vi "Find Channel Names Array.vi"(11 "Instrument Driver Method Descriptor Array":T2) -> (1 "Found?":bool, 2 "Channel List Size":i32, 3 "Channel Names":T1)   [LabVIEW 2021]
uses:
  <vilib>/myRIO/Common/Express VI Framework/typedefs/Instrument Driver Method Descriptor Array.ctl
  <vilib>/myRIO/Common/Express VI Framework/typedefs/Instrument Driver Method Descriptor.ctl
  <vilib>/myRIO/Common/Express VI Framework/typedefs/Channel Alias List.ctl
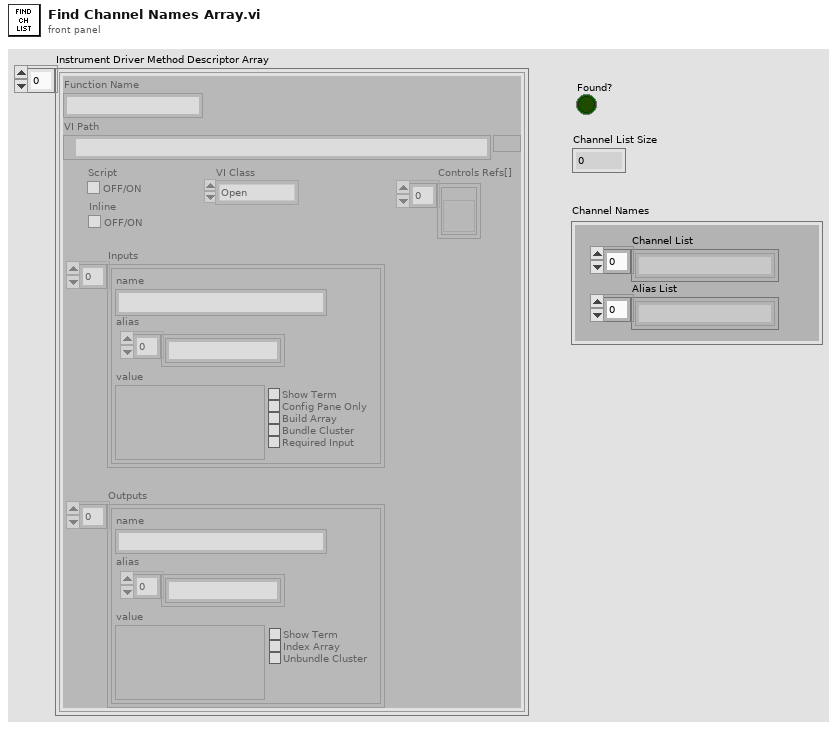
[diagram p1: front panel]
types:
  T1 = typedef "Channel Alias List.ctl" = cluster{"Channel List":string[], "Alias List":string[]}
  T2 = typedef "Instrument Driver Method Descriptor Array.ctl" = T3[]
  T3 = typedef "Instrument Driver Method Descriptor.ctl" = cluster{"Function Name":string, "VI Path":path, "Script":bool, "Inputs":cluster{"name":string, "value":variant, "Config Pane Only":bool, "Build Array":bool, "Bundle Cluster":bool, "Show Term":bool, "alias":string[], "Required Input":bool}[], "Outputs":cluster{"name":string, "value":variant, "Show Term":bool, "Index Array":bool, "Unbundle Cluster":bool, "alias":string[]}[], "VI Class":enum16{"Open", "Configure", "Data", "Manage", "Close"}, "Controls Refs[]":refnum<vi>[], "Inline":bool}
  T4 = cluster{"name":string, "value":variant, "Config Pane Only":bool, "Build Array":bool, "Bundle Cluster":bool, "Show Term":bool, "alias":string[], "Required Input":bool}[]
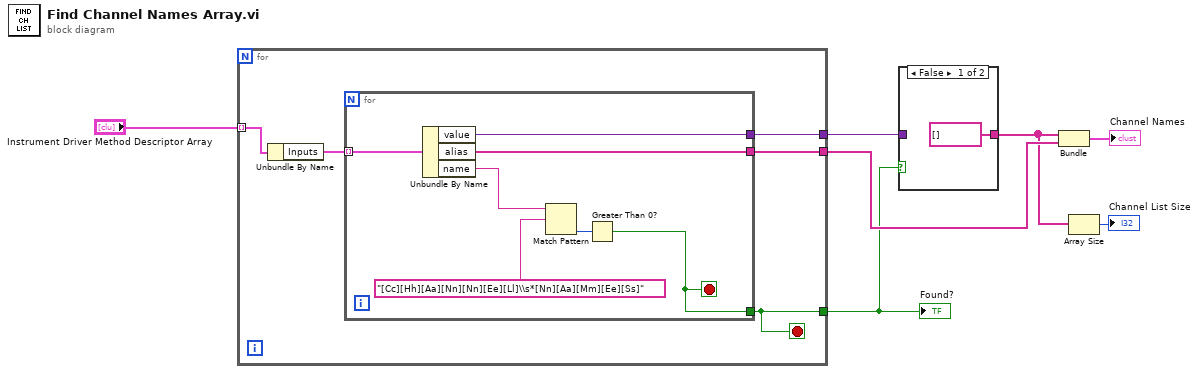
[diagram p0: block diagram]
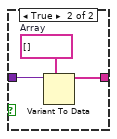
[diagram p2: hidden frame]
diagram:
  n1 = for {
    tunnel: "Instrument Driver Method Descriptor Array" -> [w12] mode=indexing
    tunnel: [w11] -> w6
    tunnel: [w10] -> w5
    tunnel: [w9] -> w1
    stop <- w9 stop-if-true
    n2 = Unbundle By Name(w12) -> ("Inputs"=w8:T4)
    n3 = for {
      tunnel: w8 -> [w16] mode=indexing
      tunnel: [w15] -> w9
      tunnel: [w14] -> w11
      tunnel: [w13] -> w10
      stop <- w15 stop-if-true
      n4 = Unbundle By Name(w16) -> ("value"=w14:variant, "alias"=w13:string[], "name"=w19:string)
      n5 = Match Pattern(string=w19, regular expression="[Cc][Hh][Aa][Nn][Nn][Ee][Ll]\\s*[Nn][Aa][Mm][Ee][Ss]") -> (offset past match=w18:i32)  [unwired: 1 in, 3 out]
      n6 = Greater Than 0?(x=w18) -> (x > 0?=w15:bool)
    }
  }
  "Found?" <- w1
  n7 = case shown="False" w1 {
    tunnel: w6 -> [_ w22]
    tunnel: [string[] [] ("Array") w21] -> w3
    frame False {
    }
    frame True {
      w23 = string[] []  # Array
      n8 = Variant To Data(type=w23, Variant=w22) -> (data=w21:string[])  [unwired: 1 in, 1 out]
    }
  }
  n9 = Bundle("Array"=w3, "alias"=w5) -> (→"Channel Names":cluster{"Array":string[], "alias":string[]})  [unwired: 1 in]
  n10 = Array Size(array=w3) -> (size(s)=→"Channel List Size":i32)
